vi "get_meas_env.vi"(10 "Stimuli":T3) -> (1 "Meas environment":T1, 2 "Load Set":T2)   [LabVIEW 2024]
doc: "Based on the stimuli cluster the VI generates the Load Set cluster and Meas environment cluster."
uses:
  ctl_stimuli_cluster.ctl
  ctl_loads_enum.ctl
  ctl_load_set_cluster.ctl
  ctl_meas_env_cluster.ctl
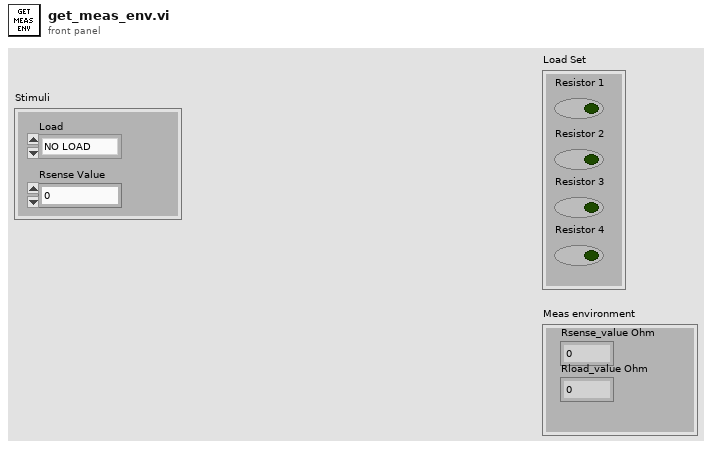
[diagram p1: front panel]
types:
  T1 = typedef "ctl_meas_env_cluster.ctl" = cluster{"Rsense_value Ohm":dbl, "Rload_value Ohm":dbl}
  T2 = typedef "ctl_load_set_cluster.ctl" = cluster{"Resistor 1":bool, "Resistor 2":bool, "Resistor 3":bool, "Resistor 4":bool}
  T3 = typedef "ctl_stimuli_cluster.ctl" = cluster{"Load":T4, "Rsense Value":dbl}
  T4 = typedef "ctl_loads_enum.ctl" = enum16{"NO LOAD", "10Ohm", "6.8Ohm", "4.7Ohm", "3.3Ohm", "2.4Ohm", "1.6Ohm", "1.3Ohm"}
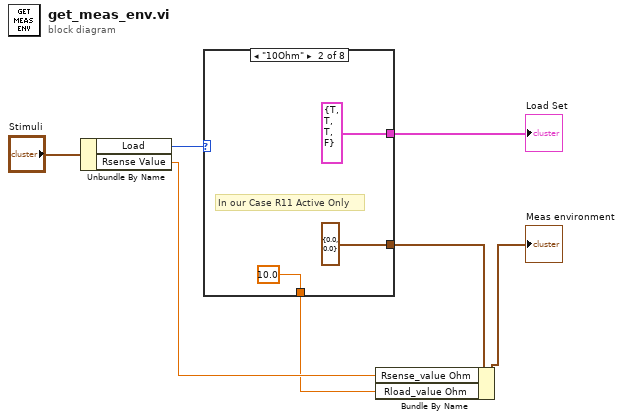
[diagram p0: block diagram]
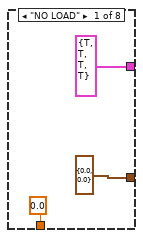
[diagram p2: hidden frame]
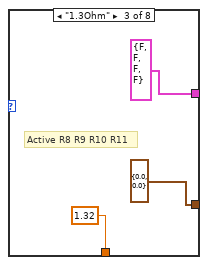
[diagram p3: hidden frame]
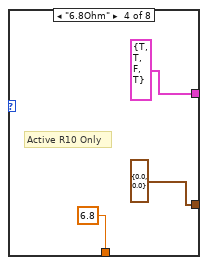
[diagram p4: hidden frame]
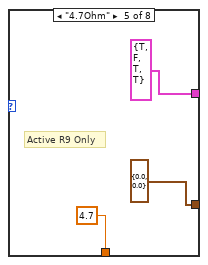
[diagram p5: hidden frame]
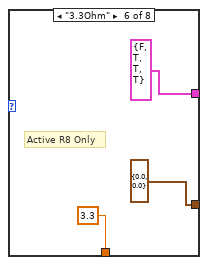
[diagram p6: hidden frame]
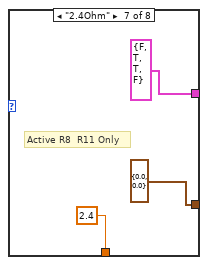
[diagram p7: hidden frame]
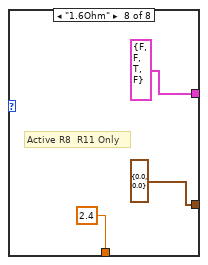
[diagram p8: hidden frame]
diagram:
  n1 = Unbundle By Name("Stimuli") -> ("Load"=w5:T4, "Rsense Value"=w2:dbl)
  n2 = case shown="\"10Ohm\"" w5 {
    tunnel: [T2 {"Resistor 1"=TRUE, "Resistor 2"=TRUE, "Resistor 3"=TRUE, "Resistor 4"=TRUE} ("Load Set") T2 {"Resistor 1"=TRUE, "Resistor 2"=TRUE, "Resistor 3"=TRUE, "Resistor 4"=FALSE} ("Load Set") T2 {"Resistor 1"=FALSE, "Resistor 2"=FALSE, "Resistor 3"=FALSE, "Resistor 4"=FALSE} ("Load Set") T2 {"Resistor 1"=TRUE, "Resistor 2"=TRUE, "Resistor 3"=FALSE, "Resistor 4"=TRUE} ("Load Set") T2 {"Resistor 1"=TRUE, "Resistor 2"=FALSE, "Resistor 3"=TRUE, "Resistor 4"=TRUE} ("Load Set") T2 {"Resistor 1"=FALSE, "Resistor 2"=TRUE, "Resistor 3"=TRUE, "Resistor 4"=TRUE} ("Load Set") T2 {"Resistor 1"=FALSE, "Resistor 2"=TRUE, "Resistor 3"=TRUE, "Resistor 4"=FALSE} ("Load Set") T2 {"Resistor 1"=FALSE, "Resistor 2"=FALSE, "Resistor 3"=TRUE, "Resistor 4"=FALSE} ("Load Set")] -> w6
    tunnel: [T1 {"Rsense_value Ohm"=0.0, "Rload_value Ohm"=0.0} ("Meas environment") T1 {"Rsense_value Ohm"=0.0, "Rload_value Ohm"=0.0} ("Meas environment") T1 {"Rsense_value Ohm"=0.0, "Rload_value Ohm"=0.0} ("Meas environment") T1 {"Rsense_value Ohm"=0.0, "Rload_value Ohm"=0.0} ("Meas environment") T1 {"Rsense_value Ohm"=0.0, "Rload_value Ohm"=0.0} ("Meas environment") T1 {"Rsense_value Ohm"=0.0, "Rload_value Ohm"=0.0} ("Meas environment") T1 {"Rsense_value Ohm"=0.0, "Rload_value Ohm"=0.0} ("Meas environment") T1 {"Rsense_value Ohm"=0.0, "Rload_value Ohm"=0.0} ("Meas environment")] -> w4
    tunnel: [0.0 ("Rload_value Ohm") 10.0 ("Rload_value Ohm") 1.32 ("Rload_value Ohm") 6.8 ("Rload_value Ohm") 4.7 ("Rload_value Ohm") 3.3 ("Rload_value Ohm") 2.4 ("Rload_value Ohm") 2.4 ("Rload_value Ohm")] -> w1
    frame "NO LOAD" {
    }
    frame "10Ohm" {
      # "In our Case R11 Active Only"
    }
    frame "1.3Ohm" {
      # "Active R8 R9 R10 R11"
    }
    frame "6.8Ohm" {
      # "Active R10 Only"
    }
    frame "4.7Ohm" {
      # "Active R9 Only"
    }
    frame "3.3Ohm" {
      # "Active R8 Only"
    }
    frame "2.4Ohm" {
      # "Active R8  R11 Only"
    }
    frame "1.6Ohm" {
      # "Active R8  R11 Only"
    }
  }
  "Load Set" <- w6
  n3 = Bundle By Name(cluster=w4, "Rsense_value Ohm"=w2, "Rload_value Ohm"=w1) -> (→"Meas environment":T1)
